vi "CS Active.vi"(7 "SPI Connection":refnum<class "SPI Connection.lvclass">, 8 "error in (no error)":errorcluster, 10 "CS Active":bool) -> (0 "error out":errorcluster)   [LabVIEW 2024, in "CTI.lvlib" / "SPI Connection.lvclass"]
uses:
  SPI Connection.lvclass
  SPI Connection.lvclass/SPI Connection.ctl
  Session/Session.lvclass
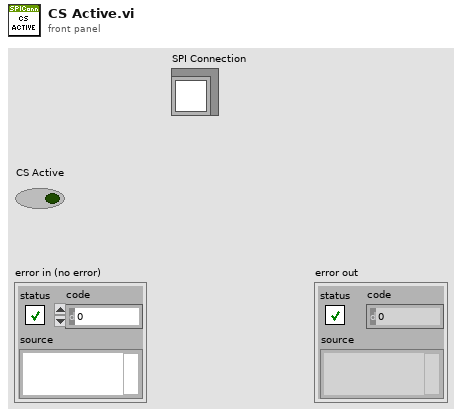
[diagram p1: front panel]
types:
  T1 = typedef "CTI.lvlib/GPIO Number.ctl" = i8
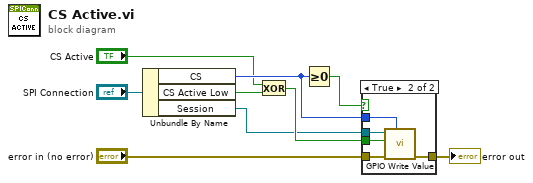
[diagram p0: block diagram]
diagram:
  n1 = Unbundle By Name("SPI Connection") -> ("CS"=w8:T1, "CS Active Low"=w6:bool, "Session"=w1:refnum<class "Session.lvclass">)
  n2 = Exclusive Or(1:w6, 2:"CS Active") -> (0:w4:bool)
  n3 = Greater Or Equal To 0?(x=w8) -> (x >= 0?=w9:bool)
  n4 = case shown="True" w9 {
    tunnel: [w10 w15] -> w3
    tunnel: w8 -> [_ w14]
    tunnel: w4 -> [_ w13]
    tunnel: w1 -> [_ w12]
    tunnel: "error in (no error)" -> [w10 w11]
    frame False {
    }
    frame True {
      n5 = call "GPIO Write Value.vi"("GPIO #"=w14, "error in (no error)"=w11, "Value"=w13, "Session in"=w12) -> ("error out"=w15:errorcluster)  [unwired: 6 in, 1 out]
    }
  }
  "error out" <- w3
